vi "Write PMT Gain.vi"(8 "error in (no error)":errorcluster, 10 "PMT Gain":refnum<k21>="PMT Gain", 11 "eCRDS in":refnum<class "eCRDS.lvclass">) -> (0 "error out":errorcluster, 3 "eCRDS out":refnum<class "eCRDS.lvclass">)   [LabVIEW 2014, in "eCRDS.lvclass"]
uses:
  eCRDS.lvclass
  eCRDS.lvclass/eCRDS.ctl
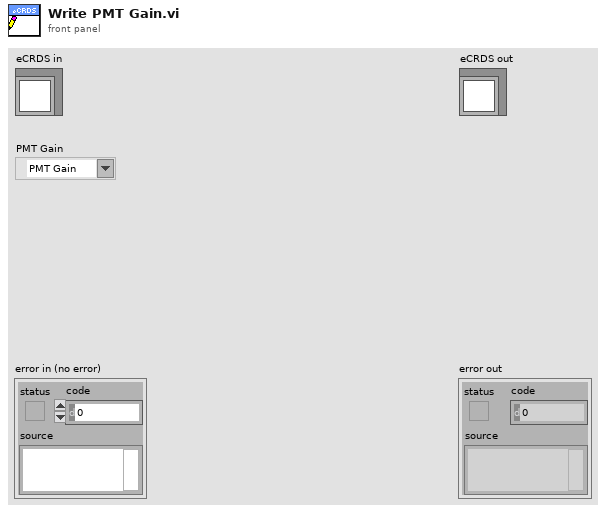
[diagram p1: front panel]
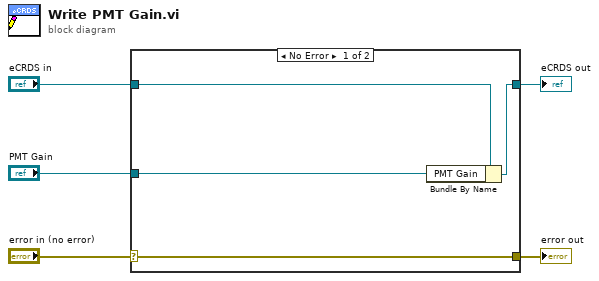
[diagram p0: block diagram]
diagram:
  n1 = case shown="No Error" "error in (no error)" {
    selector: "error in (no error)" -> [w9 w10]
    tunnel: [w9 w10] -> w4
    tunnel: [w7 w11] -> w2
    tunnel: "eCRDS in" -> [w8 w11]
    tunnel: "PMT Gain" -> [w6 _]
    frame No Error {
      n2 = Bundle By Name(cluster=w8, "PMT Gain"=w6) -> (w7:refnum<class "eCRDS.lvclass">)
    }
    frame Error {
    }
  }
  "error out" <- w4
  "eCRDS out" <- w2
